vi "scan2d_format_image.vi"(8 "error in (no error)":errorcluster, 11 "scan_panel in":refnum<class "scan_2d.lvclass">) -> (0 "error out":errorcluster, 3 "panel out":refnum<class "scan_2d.lvclass">)   [LabVIEW 2015, in "scan_2d.lvclass"]
uses:
  scan_2d.lvclass
  UI/panel_class/panel.lvclass/panel.ctl
  scan_2d.lvclass/scan_2d.ctl
  <vilib>/Utility/miscctls.llb/LVOffsetAndMultiplierTypeDef.ctl
  UI/front_panel_class/rdbu_256.ctl
  UI/panel_class/panel.lvclass
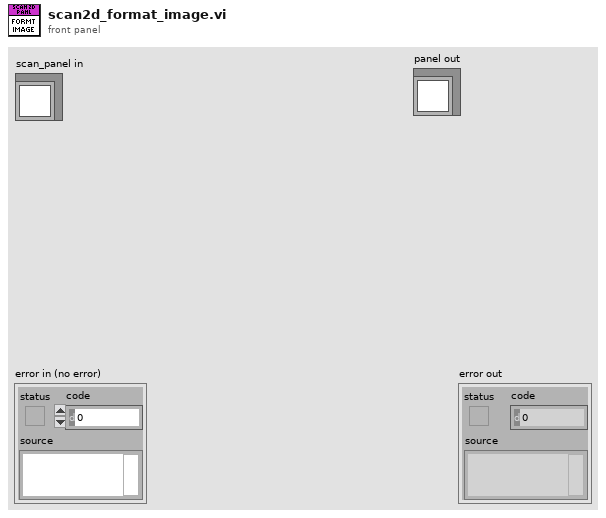
[diagram p1: front panel]
types:
  T1 = typedef "ui_plot_references.ctl" = cluster{"plots":refnum<vi>, "chart":refnum<vi>, "graph":refnum<vi>, "map":refnum<vi>, "XY Graph":refnum<vi>}
  T2 = typedef "rdbu_256.ctl" = u32[]
  T3 = typedef "LVOffsetAndMultiplierTypeDef.ctl" = cluster{"Offset":dbl, "Multiplier":dbl}
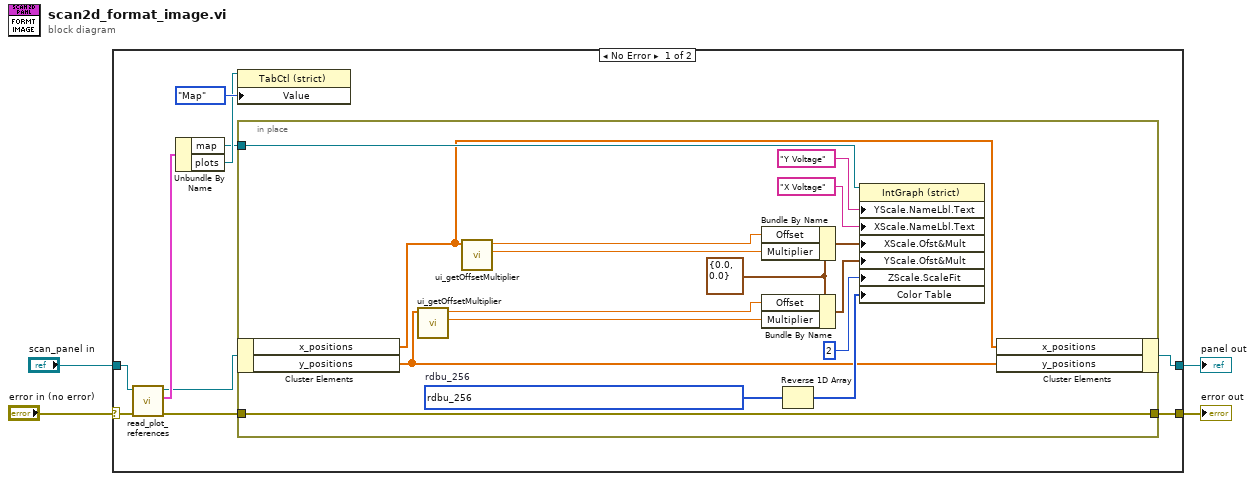
[diagram p0: block diagram]
diagram:
  n1 = case shown="No Error" "error in (no error)" {
    selector: "error in (no error)" -> [w5 w32]
    tunnel: "scan_panel in" -> [w11 w31]
    tunnel: [w8 w32] -> w3
    tunnel: [w6 w31] -> w2
    frame No Error {
      n2 = call "read_plot_references.vi"("error in (no error)"=w5, "panel in"=w11) -> ("error out"=w9:errorcluster, "plot_references"=w12:T1, "panel out"=w7:refnum<class "scan_2d.lvclass">)  [unwired: 7 in]
      n3 = Unbundle By Name(w12) -> ("map"=w10:refnum<vi>, "plots"=w13:refnum<vi>)
      n4 = property class="TabCtl (strict)"(reference=w13, "Value"=enum32{"Chart", "Graph", "Map", "XY Graph"}."Map") -> ()  [unwired: 1 in, 2 out]
      n5 = in-place {
        in-place-border: w10 -> [w29]
        in-place-border: w9 -> [w17]
        in-place-border: [w17] -> w8
        w19 = T2 [6750239, 6947103, 7143968, 7340832, 7537697, 7734561, 7931426, 8128290, 8325155, 8522019, 8718884, 8915748, 9112613, 9309221, 9506086, 9702950, 9899815, 10096679, 10293544, 10490408, 10687273, 10884137, 11081002, 11277866, 11474731, 11671595, 11671595, 11737900, 11869742, 11936047, 12067888, 12133938, 12265779, 12332085, 12463926, 12530231, 12596537, 12728378, 12794683, 12926269, 12992574, 13124415, 13190721, 13257026, 13388867, 13455173, 13587014, 13653064, 13784905, 13851210, 13983052, 14049357, 14049357, 14115663, 14181969, 14313555, 14379861, 14446168, 14512474, 14578524, 14710366, 14776672, 14842978, 14909028, 14975334, 15107177, 15173483, 15239533, 15305839, 15372145, 15503987, 15570037, 15636343, 15702650, 15768956, 15900542, 15966848, 16033154, 16033154, 16033669, 16099720, 16100234, 16101005, 16167056, 16167571, 16233621, 16234136, 16234651, 16300958, 16301472, 16301987, 16368038, 16368553, 16369067, 16435374, 16435889, 16436404, 16502454, 16502969, 16569020, 16569791, 16570305, 16636356, 16636871, 16636871, 16637129, 16637387, 16572109, 16572367, 16572881, 16573139, 16507860, 16508118, 16508376, 16508634, 16443356, 16443614, 16444128, 16444386, 16379108, 16379366, 16379624, 16379882, 16314603, 16314861, 16315375, 16315633, 16250355, 16250613, 16250871, 16250871, 16119543, 16054006, 15922678, 15856886, 15725558, 15660021, 15528693, 15462901, 15331828, 15266036, 15134708, 15068916, 14937843, 14872051, 14740723, 14674931, 14543858, 14478066, 14346738, 14281201, 14149873, 14084081, 13952753, 13887216, 13755888, 13755888, 13559023, 13427438, 13230574, 13033709, 12902124, 12705260, 12573931, 12376810, 12179945, 12048616, 11851496, 11720167, 11523302, 11326182, 11194853, 10997988, 10800867, 10669538, 10472674, 10275553, 10144224, 9947360, 9815775, 9618910, 9618910, 9421789, 9159132, 8962011, 8764890, 8567768, 8304855, 8107734, 7910613, 7647956, 7450835, 7253714, 6991056, 6793935, 6596814, 6399693, 6137036, 5939915, 5742794, 5479881, 5282760, 5085638, 4888517, 4625860, 4428739, 4428739, 4362690, 4231105, 4165056, 4033727, 3967678, 3836093, 3770044, 3703995, 3572410, 3506361, 3374776, 3308728, 3242935, 3111350, 3045301, 2913716, 2847667, 2781618, 2650033, 2584240, 2452655, 2386606, 2255021, 2188972, 2188972, 2122921, 2056870, 1990563, 1858976, 1792924, 1726617, 1660566, 1594515, 1462928, 1396877, 1330570, 1264518, 1198467, 1132160, 1066109, 934522, 868471, 802420, 736113, 670062, 538474, 472167, 406116, 340065]  # rdbu_256
        w24 = T3 {"Offset"=0.0, "Multiplier"=0.0} ("X Scale.Offset and Multiplier")
        n6 = in-place-cluster #1(w7) -> ("x_positions"=w16:dbl[], "y_positions"=w15:dbl[])
        n7 = call "ui_getOffsetMultiplier.vi"("Axis"=w15) -> ("Multiplier"=w22:dbl, "Offset"=w23:dbl)  [unwired: 9 in]
        n8 = call "ui_getOffsetMultiplier.vi"("Axis"=w16) -> ("Multiplier"=w25:dbl, "Offset"=w26:dbl)  [unwired: 9 in]
        n9 = Bundle By Name(cluster=w24, "Offset"=w26, "Multiplier"=w25) -> (w27:T3)
        n10 = Bundle By Name(cluster=w24, "Offset"=w23, "Multiplier"=w22) -> (w21:T3)
        n11 = Reverse 1D Array(array=w19) -> (reversed array=w18:T2)
        n12 = property class="IntGraph (strict)"(reference=w29, "YScale.NameLbl.Text"="Y Voltage" ("Y Scale.Name Label.Text"), "XScale.NameLbl.Text"="X Voltage" ("X Scale.Name Label.Text"), "XScale.Ofst&Mult"=w27, "YScale.Ofst&Mult"=w21, "ZScale.ScaleFit"=u8 2 ("Z Scale.Scale Fit"), "Color Table"=w18) -> ()  [unwired: 1 in, 2 out]
        n13 = in-place-cluster #1("x_positions"=w16, "y_positions"=w15) -> (w6:refnum<class "scan_2d.lvclass">)
      }
    }
    frame Error {
    }
  }
  "error out" <- w3
  "panel out" <- w2
